vi "StrNumToU8DigitArray.vi"(11 "字符串":string) -> (3 "U8数组":u8[](array[numeric]))   [LabVIEW 2012]
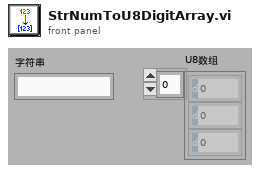
[diagram p1: front panel]
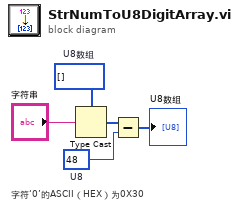
[diagram p0: block diagram]
diagram:
  w1 = u8[] []  # U8数组
  w5 = u8 48  # U8
  # "字符‘0’的ASCII（HEX）为0X30"
  n1 = Type Cast(type=w1, x="字符串") -> (*(type *) &x=w3:u8[])
  n2 = Subtract(x=w3, y=w5) -> (x-y=→"U8数组":u8[])
